vi "Monitor_AdjustFileSize.vi"(8 "Error In":errorcluster, 10 "Max File Size in Bytes":i64, 11 "Refnum In":refnum<file>) -> (0 "Error Out":errorcluster, 2 "size (in bytes)":i64, 3 "Refnum Out":refnum<file>, 5 "File Size Adjusted":bool)   [LabVIEW 2018]
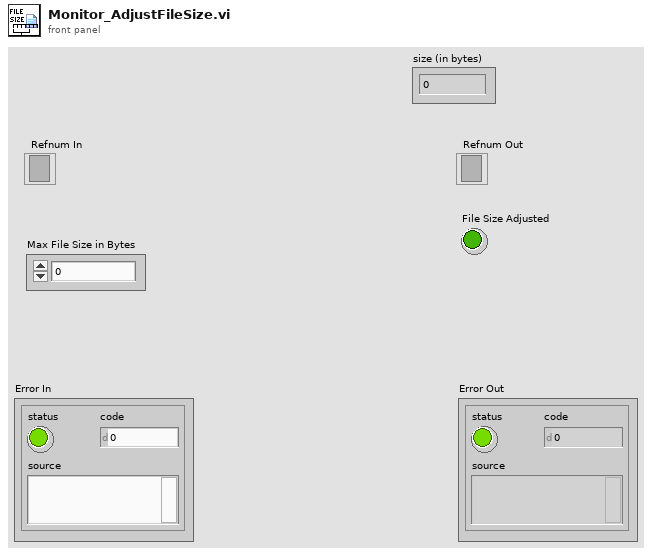
[diagram p1: front panel]
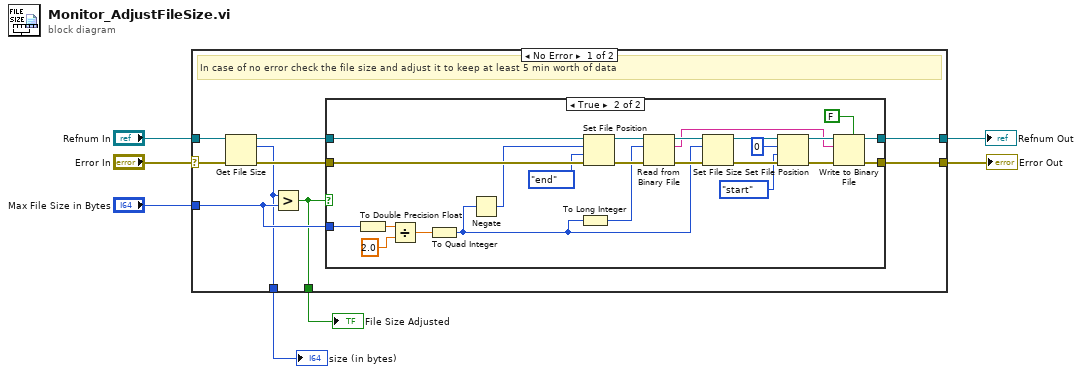
[diagram p0: block diagram]
diagram:
  n1 = case shown="No Error" "Error In" {
    selector: "Error In" -> [w16 w43]
    tunnel: "Refnum In" -> [w15 w44]
    tunnel: "Max File Size in Bytes" -> [w13 _]
    tunnel: [w11 w44] -> w4
    tunnel: [w10 w43] -> w3
    tunnel: [w9 _] -> w2
    tunnel: [w8 _] -> w1
    frame No Error {
      # "In case of no error check the file size and adjust it to keep at least 5 min worth of data"
      n2 = Get File Size(file=w15, error in=w16) -> (refnum out=w12:refnum<file>, size (in bytes)=w8:i64, 0:w14:errorcluster)
      n3 = Greater?(x=w8, y=w13) -> (0:w9:bool)
      n4 = case shown="True" w9 {
        tunnel: w14 -> [w17 w37]
        tunnel: w13 -> [_ w41]
        tunnel: w12 -> [w18 w38]
        tunnel: [w18 w20] -> w11
        tunnel: [w17 w19] -> w10
        frame False {
        }
        frame True {
          n5 = To Double Precision Float(number=w41) -> (double precision float=w42:dbl)
          n6 = Divide(x=w42, y=2.0) -> (x/y=w39:dbl)
          n7 = To Quad Integer(1:w39) -> (0:w29:i64)
          n8 = Negate(x=w29) -> (-x=w35:i64)
          n9 = To Long Integer(number=w29) -> (32bit integer=w32:i32)
          n10 = Set File Position(offset (in bytes) (0)=w35, refnum=w38, from (0:start)=enum16{"start", "end", "current"}."end", error in=w37) -> (refnum out=w34:refnum<file>, error out=w33:errorcluster)
          n11 = Read from Binary File(8:w33, 10:w32, 11:w34) -> (0:w31:errorcluster, 2:w21:string, 3:w30:refnum<file>)  [unwired: 3 in, 1 out]
          n12 = Set File Size(4:w31, 6:w29, 7:w30) -> (0:w27:errorcluster, 3:w28:refnum<file>)
          n13 = Set File Position(offset (in bytes) (0)=i64 0, refnum=w28, from (0:start)=enum16{"start", "end", "current"}."start", error in=w27) -> (refnum out=w24:refnum<file>, error out=w23:errorcluster)
          n14 = Write to Binary File(file (use dialog)=w24, data=w21, error in=w23, 5:FALSE ("prepend array or string size? (T)")) -> (refnum out=w20:refnum<file>, error out=w19:errorcluster)  [unwired: 2 in, 1 out]
        }
      }
    }
    frame Error {
      # "In case of error do nothing"
    }
  }
  "Error Out" <- w3
  "Refnum Out" <- w4
  "File Size Adjusted" <- w2
  "size (in bytes)" <- w1
